vi "Sub VI Aleator.vi"(1 "Minim":dbl, 2 "Maxim":dbl) -> (0 "X val aleatoare":dbl)   [LabVIEW 2024]
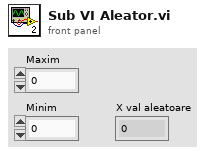
[diagram p1: front panel]
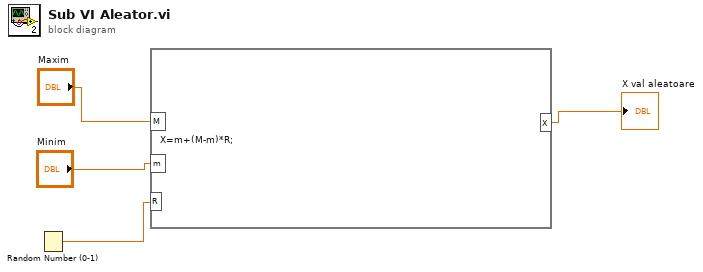
[diagram p0: block diagram]
diagram:
  n1 = Random Number (0-1)() -> (number: 0 to 1=w2:dbl)
  n2 = formula code="X=m+(M-m)*R;"("R"=w2, "m"="Minim", "M"="Maxim") -> ("X"=→"X val aleatoare":dbl)
